vi "Synapse2neurons.vi"(5 "Synapse":T2) -> (0 "Post Neuron":T1, 1 "Pre Neuron":T1)   [LabVIEW 2016]
doc: "This function gets the pre and post synaptic neurons from the input synaptic name"
uses:
  Controls/Type of Synapses.ctl
  Controls/Type of Neuron.ctl
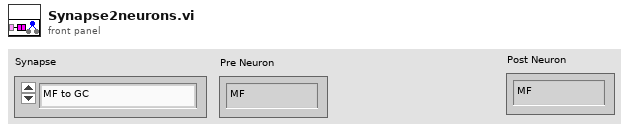
[diagram p1: front panel]
types:
  T1 = typedef "Type of Neuron.ctl" = enum16{"MF", "BA", "GO", "GC", "PC", "LU", "Glia (Dummy)"}
  T2 = typedef "Type of Synapses.ctl" = enum16{"MF to GC", "GO to GC", "GC to GO", "MF to GO", "GC to PC", "GC to BA", "PC to BA", "BA to PC", "BA to GO"}
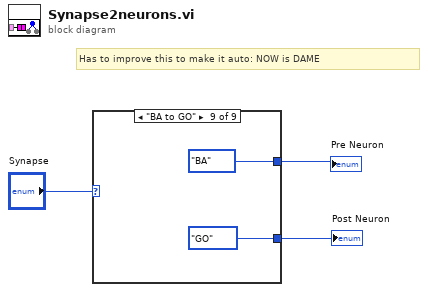
[diagram p0: block diagram]
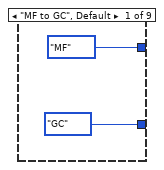
[diagram p2: hidden frame]
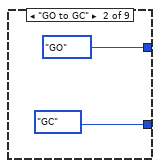
[diagram p3: hidden frame]
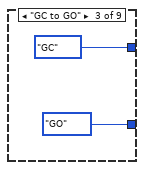
[diagram p4: hidden frame]
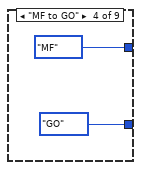
[diagram p5: hidden frame]
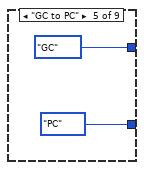
[diagram p6: hidden frame]
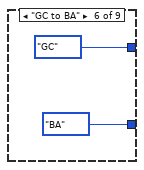
[diagram p7: hidden frame]
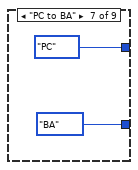
[diagram p8: hidden frame]
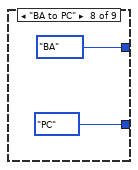
[diagram p9: hidden frame]
diagram:
  # "Has to improve this to make it auto: NOW is DAME"
  n1 = case shown="\"BA to GO\"" "Synapse" {
    tunnel: [Type_of_Neuron."MF" ("Pre Neuron") Type_of_Neuron."GO" ("Pre Neuron") Type_of_Neuron."GC" ("Pre Neuron") Type_of_Neuron."MF" ("Pre Neuron") Type_of_Neuron."GC" ("Pre Neuron") Type_of_Neuron."GC" ("Pre Neuron") Type_of_Neuron."PC" ("Pre Neuron") Type_of_Neuron."BA" ("Pre Neuron") Type_of_Neuron."BA" ("Pre Neuron")] -> w2
    tunnel: [Type_of_Neuron."GC" ("Pre Neuron") Type_of_Neuron."GC" ("Pre Neuron") Type_of_Neuron."GO" ("Pre Neuron") Type_of_Neuron."GO" ("Pre Neuron") Type_of_Neuron."PC" ("Pre Neuron") Type_of_Neuron."BA" ("Pre Neuron") Type_of_Neuron."BA" ("Pre Neuron") Type_of_Neuron."PC" ("Pre Neuron") Type_of_Neuron."GO" ("Pre Neuron")] -> w1
    frame "MF to GC", Default {
    }
    frame "GO to GC" {
    }
    frame "GC to GO" {
    }
    frame "MF to GO" {
    }
    frame "GC to PC" {
    }
    frame "GC to BA" {
    }
    frame "PC to BA" {
    }
    frame "BA to PC" {
    }
    frame "BA to GO" {
    }
  }
  "Pre Neuron" <- w2
  "Post Neuron" <- w1
